vi "lr2.vi"() -> ()   [LabVIEW 2012]
panel:
  out "?":bool
  out "Max":bool
  out "Min":bool
  out "Meter":dbl(knob) scale=-25.0..25.0
  in  "Num max":dbl
  in  "Num min":dbl
  in  "Time reg":dbl(slide) scale=0.0..300.0
  out "Waveform  2":dbl(graph)
  out "Waveform 1":dbl[](graph)
  in  "stop":bool
  in  "?":bool
  in  "X2":dbl(knob) scale=-10.0..10.0
  in  "X1":dbl(knob) scale=-10.0..10.0
  in  "U2":dbl(slide) scale=-10.0..10.0
  in  "U1":dbl(slide) scale=-10.0..10.0
  # "1"
  # "2"
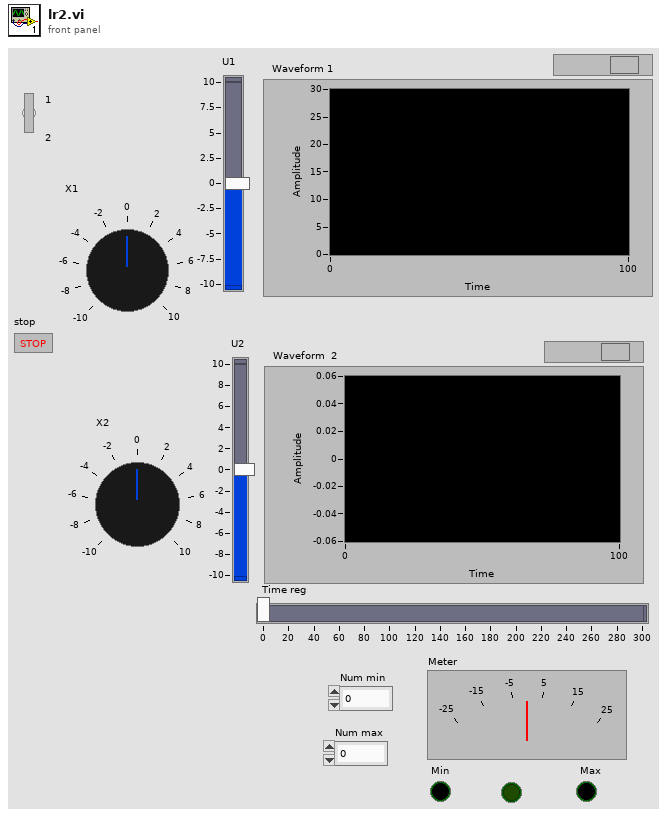
[diagram p1: front panel]
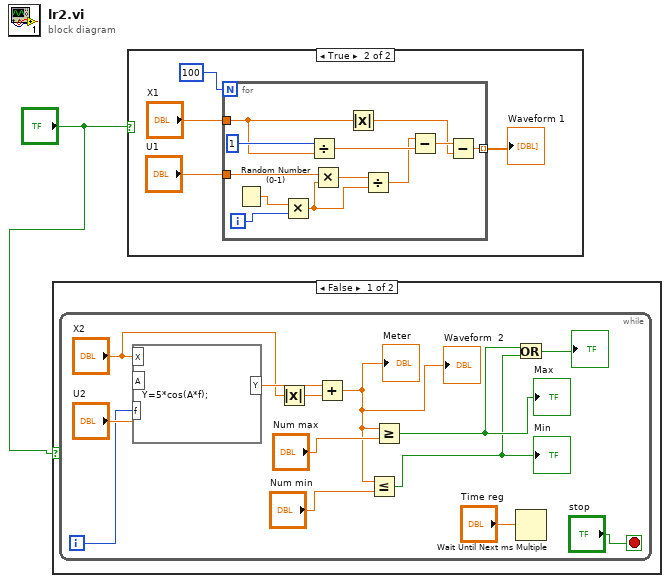
[diagram p0: block diagram]
diagram:
  n1 = case shown="False" "?" {
    frame False {
      n2 = while {
        i -> [w6]
        stop <- "stop" stop-if-true
        n3 = formula code="Y=5*cos(A*f);"("A"="U2", "f"=w6, "X"="X2") -> ("Y"=w5:dbl)
        n4 = Absolute Value(x="X2") -> (abs(x)=w3:dbl)
        n5 = Add(x=w5, y=w3) -> (x+y=w4:dbl)
        "Meter" <- w4
        "Waveform  2" <- w4
        n6 = Less Or Equal?(x=w4, y="Num min") -> (x <= y?=w10:bool)
        "Min" <- w10
        n7 = Greater Or Equal?(x=w4, y="Num max") -> (x >= y?=w11:bool)
        "Max" <- w11
        n8 = Or(x=w11, y=w10) -> (x .or. y?=→"?":bool)
        n9 = Wait Until Next ms Multiple(millisecond multiple="Time reg") -> ()  [unwired: 1 out]
      }
    }
    frame True {
    }
  }
  n10 = case shown="True" "?" {
    frame False {
    }
    frame True {
      n11 = for {
        N: 100 -> [_]
        tunnel: [w19] -> w17 mode=indexing
        tunnel: "U1" -> [w28]
        tunnel: "X1" -> [w24]
        i -> [w30]
        n12 = Random Number (0-1)() -> (number: 0 to 1=w29:dbl)
        n13 = Multiply(x=w29, y=w30) -> (x*y=w26:dbl)
        n14 = Divide(x=1, y=w24) -> (x/y=w23:dbl)
        n15 = Multiply(x=w28, y=w26) -> (x*y=w27:dbl)
        n16 = Absolute Value(x=w24) -> (abs(x)=w20:dbl)
        n17 = Divide(x=w27, y=w26) -> (x/y=w22:dbl)
        n18 = Subtract(x=w22, y=w23) -> (x-y=w21:dbl)
        n19 = Subtract(x=w21, y=w20) -> (x-y=w19:dbl)
      }
      "Waveform 1" <- w17
    }
  }
